vi "keypad project_0.vi"() -> ()   [LabVIEW 2015]
uses:
  <vilib>/myRIO/Instrument Drivers/Onboard IO/DIO/typedefs/DIO Reference.ctl
  <vilib>/myRIO/Common/Instrument Driver Framework/Utilities/typedefs/myRIO Generic Hardware Reference.ctl
  <vilib>/myRIO/Common/Instrument Driver Framework/Utilities/typedefs/Hardware Version Enum.ctl
  <vilib>/myRIO/Common/Instrument Driver Framework/Utilities/typedefs/myRIO v1.0 Reference.ctl
  <vilib>/myRIO/Common/Instrument Driver Framework/Utilities/typedefs/Generic FPGA Reference.ctl
  <vilib>/myRIO/Common/Instrument Driver Framework/myRIO v1.0/DIO/typedefs/DIO Channels List.ctl
  <vilib>/myRIO/Common/Instrument Driver Framework/myRIO v1.0/DIO/typedefs/DIO Channels Enum.ctl
  <vilib>/userdefined/High Color/nirio_resource_hc.ctl
  <vilib>/myRIO/Common/Instrument Driver Framework/Utilities/vis/Is FPGA Ref Available.vi
  <vilib>/myRIO/Common/Instrument Driver Framework/myRIO v1.0/DIO/vis/myRIO v1.1 Open DIO.vi
  <vilib>/myRIO/Common/Instrument Driver Framework/Utilities/vis/Validate Channels.vi
  <vilib>/myRIO/Common/Instrument Driver Framework/myRIO v1.0/DIO/vis/myRIO v1.0 Reserve DIO.vi
  <vilib>/myRIO/Common/Instrument Driver Framework/myRIO v1.0/UART/vis/myRIO v1.0 Close UART.vi
  <vilib>/myRIO/Common/Instrument Driver Framework/myRIO v1.0/Resource Manager/vis/myRIO v1.0 Reserve Channel List.vi
  <vilib>/myRIO/Common/Instrument Driver Framework/myRIO v1.0/DIO/vis/myRIO v1.0 Build MUX Configuration DIO.vi
  <vilib>/myRIO/Common/Instrument Driver Framework/myRIO v1.0/Resource Manager/vis/myRIO v1.0 Reserve Channel.vi
  <vilib>/myRIO/Common/Instrument Driver Framework/myRIO v1.0/Resource Manager/vis/myRIO v1.0 Unreserve Channel.vi
  <vilib>/myRIO/Common/Instrument Driver Framework/myRIO v1.0/Resource Manager/vis/myRIO v1.0 Create Configuration List.vi
  <vilib>/myRIO/Common/Instrument Driver Framework/myRIO v1.0/Resource Manager/vis/myRIO v1.0 Build Mutex Name.vi
  <vilib>/Utility/VariantDataType/GetNumericInfo.vi
  <vilib>/Utility/error.llb/Error Cluster From Error Code.vi
  <vilib>/myRIO/Common/Instrument Driver Framework/myRIO v1.0/myRIO v1.1 Open.vi
  <vilib>/myRIO/Common/Instrument Driver Framework/Utilities/vis/IO Manager.vi
  <vilib>/myRIO/Common/Instrument Driver Framework/Utilities/vis/Configuration Manager.vi
  <vilib>/myRIO/Common/Instrument Driver Framework/myRIO v1.0/Resource Manager/vis/myRIO v1.0 Configure IO.vi
  <vilib>/myRIO/Common/Instrument Driver Framework/myRIO v1.0/myRIO v1.0 Close.vi
  <vilib>/myRIO/Common/Instrument Driver Framework/myRIO v1.0/DIO/vis/myRIO v1.0 Read DIO.vi
  <vilib>/myRIO/Common/Instrument Driver Framework/myRIO v1.0/DIO/vis/myRIO v1.0 Write DIO.vi
  <vilib>/myRIO/Instrument Drivers/Onboard IO/DIO/vis/Smart Open.vi
  <vilib>/myRIO/Common/Instrument Driver Framework/Utilities/vis/FPGA Ref Manager.vi
  <vilib>/myRIO/Common/Instrument Driver Framework/myRIO v1.0/myRIO v1.0 Reset FPGA.vi
  <vilib>/myRIO/Common/Instrument Driver Framework/myRIO v1.0/IRQ/vis/myRIO v1.0 IRQ Info FGV.vi
  <vilib>/myRIO/Common/Instrument Driver Framework/myRIO v1.0/IRQ/vis/myRIO v1.0 Timer IRQ Info FGV.vi
  <vilib>/myRIO/Common/Instrument Driver Framework/myRIO v1.0/IRQ/vis/myRIO v1.0 ISR Agent.vi
  <vilib>/myRIO/Express VI/Onboard IO/DO/DO Express VI.xnode
  <vilib>/myRIO/Instrument Drivers/Onboard IO/DIO/vis/myRIO DIO Open.xnode
  <vilib>/myRIO/Instrument Drivers/Onboard IO/DIO/DIO.lvlib
  <vilib>/myRIO/Instrument Drivers/Utilities/Utilities.lvlib
panel:
  out "Array":errorcluster[](array[cluster])
  in  "Tab Control":enum32{"Page 1", "Page 2"}(tab)
  out "Scan":bool[](array[boolean])
  out "Keypad buttons":bool[][](array[boolean])
  in  "[ESC]":bool
  # "Keypad project"
  # "Pardeep kumar"
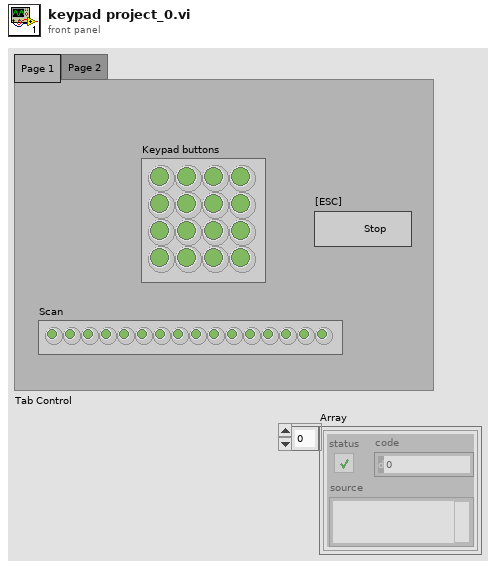
[diagram p1: front panel]
types:
  T1 = typedef "DIO.lvlib/DIO Reference.ctl" = cluster{"myRIO Reference":T2, "DIO Channels List":T6}
  T2 = typedef "myRIO Generic Hardware Reference.ctl" = cluster{"myRIO Model":T3, "myRIO Hardware Reference":T4}
  T3 = typedef "Hardware Version Enum.ctl" = enum16{"Unknown", "myRIO-1900", "myRIO-1950", "roboRIO"}
  T4 = typedef "myRIO v1.0 Reference.ctl" = cluster{"Generic FPGA Reference":T5, "Allow multiple opens":bool}
  T5 = typedef "Generic FPGA Reference.ctl" = refnum<k20>
  T6 = typedef "DIO Channels List.ctl" = T7[]
  T7 = typedef "DIO Channels Enum.ctl" = enum16{"Not Connected", "C/DIO0", "C/DIO1", "C/DIO2", "C/DIO3", "C/DIO4", "C/DIO5", "C/DIO6", "C/DIO7", "A/DIO0", "A/DIO1", "A/DIO2", "A/DIO3", "A/DIO4", "A/DIO5", "A/DIO6", "A/DIO7", "A/DIO8", "A/DIO9", "A/DIO10", "A/DIO11", "A/DIO12", "A/DIO13", "A/DIO14", "A/DIO15", "B/DIO0", "B/DIO1", "B/DIO2", "B/DIO3", "B/DIO4", "B/DIO5", "B/DIO6", "B/DIO7", "B/DIO8", "B/DIO9", "B/DIO10", "B/DIO11", "B/DIO12", "B/DIO13", "B/DIO14", "B/DIO15", "LED0", "LED1", "LED2", "LED3", "Button0", "DIO/DIO0", "DIO/DIO1", "DIO/DIO2", "DIO/DIO3", "DIO/DIO4", "DIO/DIO5", "DIO/DIO6", "DIO/DIO7", "DIO/DIO8", "DIO/DIO9", "SPI/CS0", "SPI/CS1", "SPI/CS2", "SPI/CS3", "LED RADIO (Green)", "LED RADIO (Red)", "LED COMM (Green)", "LED COMM (Red)", "LED MODE (Green)", "LED MODE (Red)"}
  T8 = typedef "nirio_resource_hc.ctl" = tag
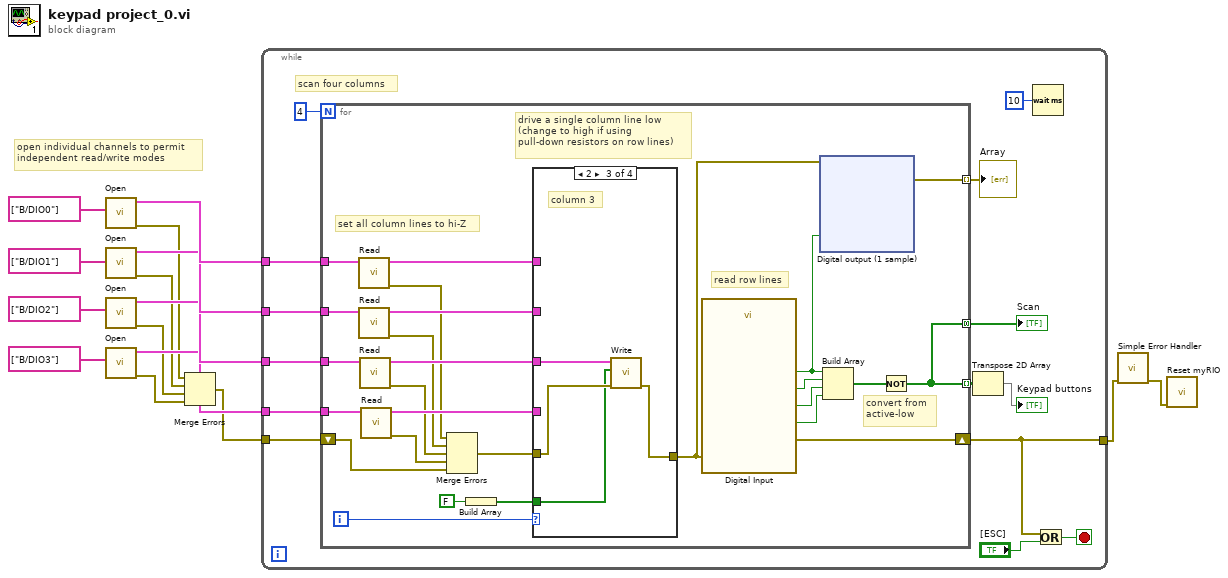
[diagram p0: block diagram]
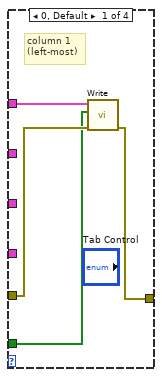
[diagram p2: hidden frame]
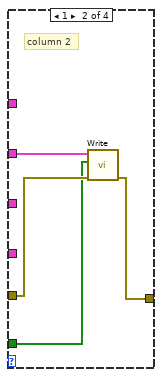
[diagram p3: hidden frame]
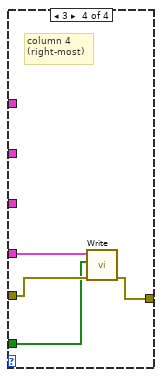
[diagram p4: hidden frame]
diagram:
  # "open individual channels to permit\nindependent read/write modes"
  n1 = call <vilib>:"Open.vi"("Channel Names"=tag[] ["B/DIO0"]) -> ("error out"=w5:errorcluster, "DIO Ref Out"=w9:T1)  [unwired: 9 in]
  n2 = call <vilib>:"Open.vi"("Channel Names"=tag[] ["B/DIO1"]) -> ("error out"=w4:errorcluster, "DIO Ref Out"=w8:T1)  [unwired: 9 in]
  n3 = call <vilib>:"Open.vi"("Channel Names"=tag[] ["B/DIO2"]) -> ("error out"=w3:errorcluster, "DIO Ref Out"=w7:T1)  [unwired: 9 in]
  n4 = call <vilib>:"Open.vi"("Channel Names"=tag[] ["B/DIO3"]) -> ("error out"=w2:errorcluster, "DIO Ref Out"=w6:T1)  [unwired: 9 in]
  n5 = Merge Errors "Merge Errors"(w5, w4, w3, w2) -> (w1:errorcluster)
  n6 = while {
    tunnel: [w25] -> w15
    tunnel: w9 -> [w22]
    tunnel: w8 -> [w21]
    tunnel: w7 -> [w20]
    tunnel: w6 -> [w19]
    tunnel: w1 -> [w18]
    stop <- w29 stop-if-true
    # "scan four columns"
    n7 = for {
      N: 4 -> [_]
      tunnel: [w50] -> w24 mode=indexing
      shift-right: [w32] -> w25
      shift-left: w18 -> [w37]
      tunnel: [w50] -> w17 mode=concatenating
      tunnel: w22 -> [w49]
      tunnel: w21 -> [w46]
      tunnel: w20 -> [w47]
      tunnel: w19 -> [w48]
      tunnel: [w31] -> w16 mode=indexing
      i -> [w55]
      # "convert from\nactive-low"
      # "set all column lines to hi-Z"
      # "read row lines"
      # "drive a single column line low\n(change to high if using \npull-down resistors on row lines)"
      n8 = call <vilib>:"Read.vi"("DIO Ref In"=w49) -> ("error out"=w41:errorcluster, "DIO Ref Out"=w45:T1)  [unwired: 8 in, 1 out]
      n9 = call <vilib>:"Read.vi"("DIO Ref In"=w46) -> ("error out"=w40:errorcluster, "DIO Ref Out"=w44:T1)  [unwired: 8 in, 1 out]
      n10 = call <vilib>:"Read.vi"("DIO Ref In"=w47) -> ("error out"=w39:errorcluster, "DIO Ref Out"=w43:T1)  [unwired: 8 in, 1 out]
      n11 = call <vilib>:"Read.vi"("DIO Ref In"=w48) -> ("error out"=w38:errorcluster, "DIO Ref Out"=w42:T1)  [unwired: 8 in, 1 out]
      n12 = Merge Errors(w41, w40, w39, w38, w37) -> (w36:errorcluster)
      n13 = Build Array "Build Array"(FALSE) -> (w34:bool[])
      n14 = case shown="2" w55 {
        tunnel: w45 -> [w94 _ _ _]
        tunnel: w44 -> [_ w98 _ _]
        tunnel: w43 -> [_ _ w102 _]
        tunnel: w42 -> [_ _ _ w106]
        tunnel: [w93 w97 w101 w105] -> w33
        tunnel: w36 -> [w92 w96 w100 w104]
        tunnel: w34 -> [w91 w95 w99 w103]
        frame 0, Default {
          # "column 1\n(left-most)"
          n15 = call <vilib>:"Write.vi"("error in (no error)"=w92, "Values"=w91, "DIO Ref In"=w94) -> ("error out"=w93:errorcluster)  [unwired: 6 in, 1 out]
        }
        frame 1 {
          # "column 2"
          n16 = call <vilib>:"Write.vi"("error in (no error)"=w96, "Values"=w95, "DIO Ref In"=w98) -> ("error out"=w97:errorcluster)  [unwired: 6 in, 1 out]
        }
        frame 2 {
          # "column 3"
          n17 = call <vilib>:"Write.vi"("error in (no error)"=w100, "Values"=w99, "DIO Ref In"=w102) -> ("error out"=w101:errorcluster)  [unwired: 6 in, 1 out]
        }
        frame 3 {
          # "column 4\n(right-most)"
          n18 = call <vilib>:"Write.vi"("error in (no error)"=w104, "Values"=w103, "DIO Ref In"=w106) -> ("error out"=w105:errorcluster)  [unwired: 6 in, 1 out]
        }
      }
      n19 = call "Digital Input"("error in (no error)"=w33) -> ("B/DIO4 (Pin 19)"=w30:bool, "B/DIO5 (Pin 21)"=w54:bool, "B/DIO6 (Pin 23)"=w53:bool, "B/DIO7 (Pin 25)"=w52:bool, "error out"=w32:errorcluster)  [unwired: 22 in]
      n20 = xnode "Digital output (1 sample)"("A/DIO0 (Pin 11)"=w30, "error in (no error)"=w33) -> ("error out"=w31:errorcluster)
      n21 = Build Array "Build Array"(w30, w54, w53, w52) -> (w51:bool[])
      n22 = Not(x=w51) -> (.not. x?=w50:bool[])
    }
    "Scan" <- w17
    "Array" <- w16
    n23 = Transpose 2D Array(2D array=w24) -> (transposed array=→"Keypad buttons":bool[][])
    n24 = Wait (ms)(milliseconds to wait=u32 10) -> ()  [unwired: 1 out]
    n25 = Or(x=w25, y="[ESC]") -> (x .or. y?=w29:bool)
  }
  n26 = call <vilib>:"Simple Error Handler.vi"("error in (no error)"=w15) -> ("error out"=w14:errorcluster)  [unwired: 4 in, 4 out]
  n27 = call <vilib>:"Reset myRIO.vi"("error in (no error)"=w14) -> ()  [unwired: 10 in, 1 out]
